vi "Base64_Decode.vi"(10 "error in (no error)":errorcluster, 11 "Base64 String":string) -> (2 "error out":errorcluster, 3 "Decoded String":string)   [LabVIEW 2013, in "Serializer.Base64.lvclass"]
uses:
  Serializer.Base64.lvclass
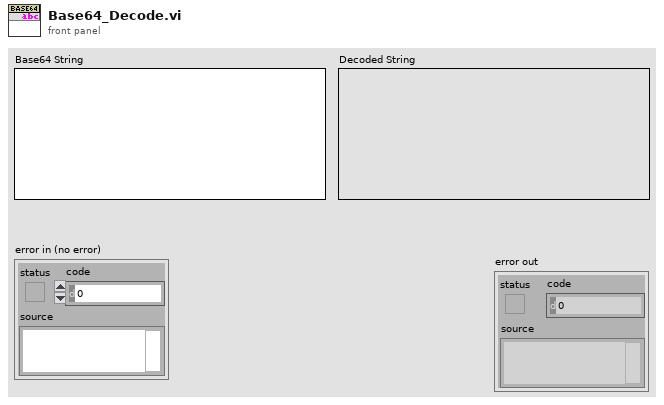
[diagram p1: front panel]
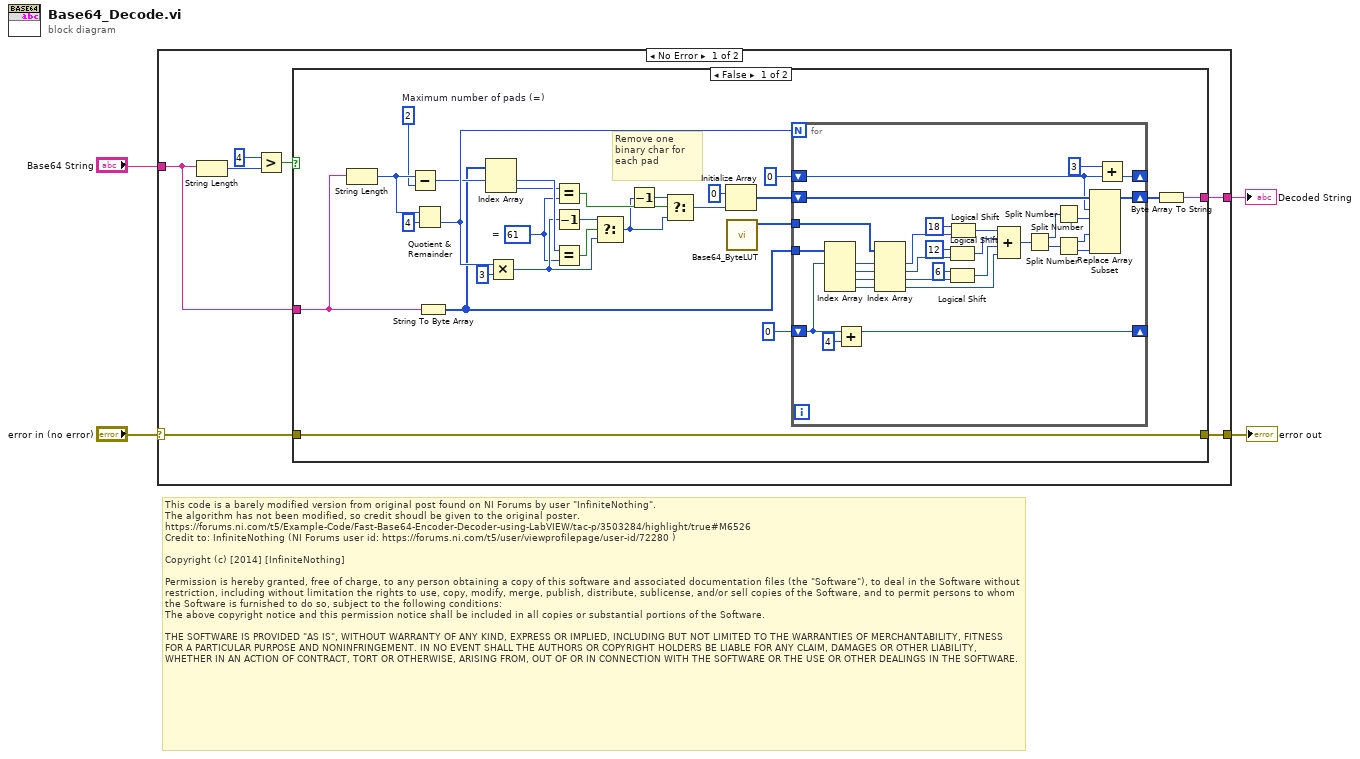
[diagram p0: block diagram]
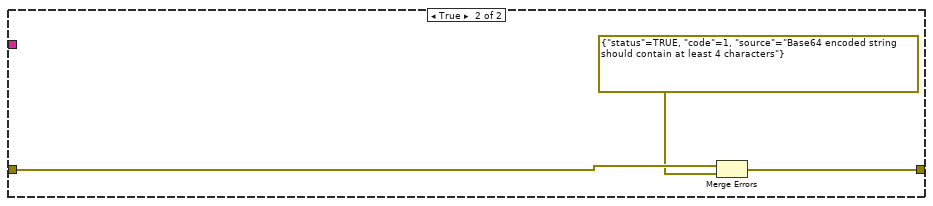
[diagram p2: hidden frame]
diagram:
  # "This code is a barely modified version from original post found on NI Forums by user \"InfiniteNothing\".\nThe algorithm has not been modified, so credit shoudl be given to the original poster.\nhttps://forums.ni.com/t5/Example-Code/Fast-Base64-Encoder-Decoder-using-LabVIEW/tac-p/3503284/highlight/true#M6526\nCredit to: InfiniteNothing (NI Forums user id: https://forums.ni.com/t5/user/viewprofilepage/user-id/72280 )\n\nCopyright (c) [2014] [InfiniteNothing]\n\nPermission is hereby granted, free of charge, to any person obtaining a copy of this software and associated documentation files (the \"Software\"), to deal in the Software without restriction, including without limitation the rights to use, copy, modify, merge, publish, distribute, sublicense, and/or sell copies of the Software, and to permit persons to whom the Software is furnished to do so, subject to the following conditions:\nThe above copyright notice and this permission notice shall be included in all copies or substantial portions of the Software.\n\nTHE SOFTWARE IS PROVIDED \"AS IS\", WITHOUT WARRANTY OF ANY KIND, EXPRESS OR IMPLIED, INCLUDING BUT NOT LIMITED TO THE WARRANTIES OF MERCHANTABILITY, FITNESS FOR A PARTICULAR PURPOSE AND NONINFRINGEMENT. IN NO EVENT SHALL THE AUTHORS OR COPYRIGHT HOLDERS BE LIABLE FOR ANY CLAIM, DAMAGES OR OTHER LIABILITY, WHETHER IN AN ACTION OF CONTRACT, TORT OR OTHERWISE, ARISING FROM, OUT OF OR IN CONNECTION WITH THE SOFTWARE OR THE USE OR OTHER DEALINGS IN THE SOFTWARE."
  n1 = case shown="No Error" "error in (no error)" {
    selector: "error in (no error)" -> [w6 w71]
    tunnel: [w9 _] -> w2
    tunnel: "Base64 String" -> [w8 _]
    tunnel: [w5 w71] -> w1
    frame No Error {
      n2 = String Length(string=w8) -> (length=w11:i32)
      n3 = Greater?(x=4 ("y"), y=w11) -> (0:w7:bool)
      n4 = case shown="False" w7 {
        tunnel: [w17 _] -> w9
        tunnel: w8 -> [w16 _]
        tunnel: w6 -> [w15 w70]
        tunnel: [w15 w68] -> w5
        frame False {
          w14 = u8 61  # =
          w29 = 2  # Maximum number of pads (=)
          # "Remove one binary char for each pad"
          n5 = String Length(string=w16) -> (length=w30:i32)
          n6 = Subtract(x=w30, y=w29) -> (x-y=w28:i32)
          n7 = Quotient & Remainder(x=w30, y=4 ("U64 Chars")) -> (floor(x/y)=w34:i32)  [unwired: 1 out]
          n8 = String To Byte Array(string=w16) -> (unsigned byte array=w12:u8[])
          n9 = Index Array(array=w12, index #1=w28) -> (element #1=w27:u8, element #2=w26:u8)  [unwired: 1 in]
          n10 = Multiply(x=w34, y=3 ("Binary chars")) -> (x*y=w20:i32)
          n11 = Equal?(x=w26, y=w14) -> (x = y?=w22:bool)
          n12 = Decrement(x=w20) -> (x-1=w21:i32)
          n13 = Equal?(x=w27, y=w14) -> (x = y?=w24:bool)
          n14 = Select(t=w21, s=w24, f=w20) -> (s? t:f=w19:i32)
          n15 = Decrement(x=w19) -> (x-1=w18:i32)
          n16 = Select(t=w18, s=w22, f=w19) -> (s? t:f=w23:i32)
          n17 = Initialize Array(u8 0 ("element"), w23) -> (w37:u8[])
          n18 = call "Base64_ByteLUT.vi"() -> ("U8 LUT"=w13:u32[])  [unwired: 11 in]
          n19 = for {
            N: w34 -> [_]
            tunnel: w12 -> [w62]
            shift-right: [w60] -> _
            shift-left: 0 ("B64 Index") -> [w61]
            shift-right: [w56] -> _
            shift-left: 0 ("Binary Index") -> [w55]
            shift-right: [w58] -> w25
            shift-left: w37 -> [w59]
            tunnel: w13 -> [w38]
            n20 = Index Array(array=w62, index #1=w61) -> (element #1=w46:u8, element #2=w45:u8, element #3=w44:u8, element #4=w43:u8)  [unwired: 3 in]
            n21 = Add(x=w61, y=4 ("B64s per 3 U8s")) -> (x+y=w60:i32)
            n22 = Index Array(array=w38, index #1=w46, index #2=w45, index #3=w44, index #4=w43) -> (element #1=w42:u32, element #2=w41:u32, element #3=w40:u32, element #4=w39:u32)
            n23 = Logical Shift(y=12, x=w41) -> (x << y=w49:u32)
            n24 = Logical Shift(y=6, x=w40) -> (x << y=w48:u32)
            n25 = Logical Shift(y=18, x=w42) -> (x << y=w50:u32)
            n26 = Compound Arithmetic op=ADD(w50, w49, w48, w39) -> (w47:u32)
            n27 = Split Number(x=w47) -> (hi(x)=w66:u16, lo(x)=w67:u16)
            n28 = Split Number(x=w66) -> (lo(x)=w65:u8)  [unwired: 1 out]
            n29 = Split Number(x=w67) -> (hi(x)=w64:u8, lo(x)=w63:u8)
            n30 = Replace Array Subset(array=w59, new element #1=w65, index #1=w55, new element #2=w64, new element #3=w63) -> (w58:u8[])  [unwired: 2 in]
            n31 = Add(x=3 ("Binary Chars per 4 B64s"), y=w55) -> (x+y=w56:i32)
          }
          n32 = Byte Array To String(unsigned byte array=w25) -> (string=w17:string)
        }
        frame True {
          n33 = Merge Errors(w70, errorcluster {"status"=TRUE, "code"=1, "source"="Base64 encoded string should contain at least 4 characters"} ("error in")) -> (w68:errorcluster)
        }
      }
    }
    frame Error {
    }
  }
  "Decoded String" <- w2
  "error out" <- w1
